vi "TDMS2TDMGlobalLog.vi"(0 "Original Name":string, 1 "New Name":string, 2 "Log File Path":path, 3 "Original Datatype":string, 4 "New Datatype":string, 5 "error in (no error)":errorcluster, 6 "Str Refnum":refnum<vi>, 8 "Operation":T1) -> (19 "error out":errorcluster)   [LabVIEW 2020]
uses:
  <vilib>/Utility/tdmsutil.llb/TDMS2TDMLogOperation.ctl
  <vilib>/Utility/error.llb/DialogType.ctl
  Instance           5 25Saved   TDMS2TDMGlobalLog .vi
  Instance           3 25Saved   TDMS2TDMGlobalLog .vi
  Instance           2 25Saved   TDMS2TDMGlobalLog .vi
  Instance           1 25Saved   TDMS2TDMGlobalLog .vi
  Instance           4 25Saved   TDMS2TDMGlobalLog .vi
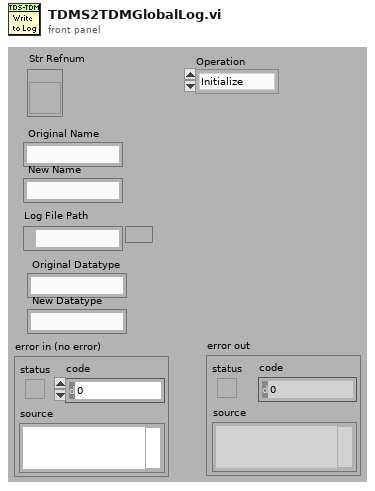
[diagram p1: front panel]
types:
  T1 = typedef "TDMS2TDMLogOperation.ctl" = enum16{"Initialize", "Data Conversion", "Name Conversion", "Write Log File"}
  T2 = enum16{"open", "replace", "create", "open or create", "replace or create", "replace or create with confirmation"}
  T3 = typedef "DialogType.ctl" = u16
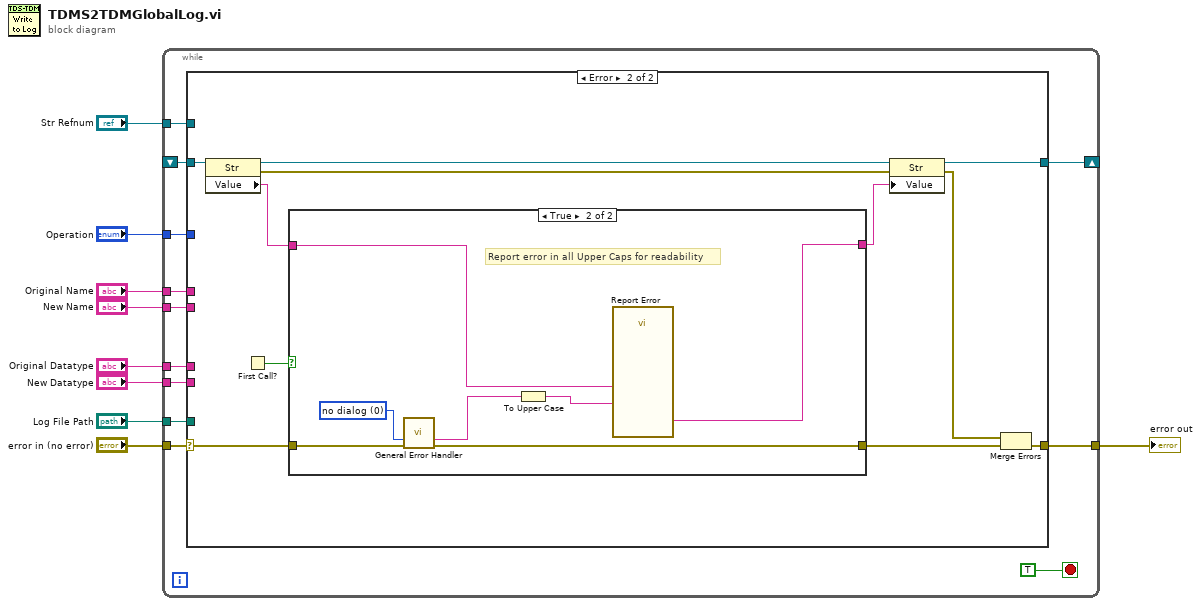
[diagram p0: block diagram]
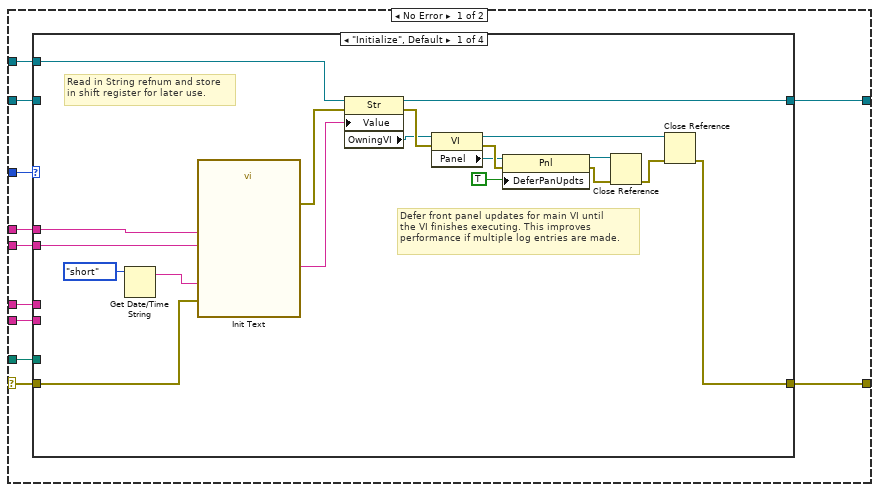
[diagram p2: hidden frame]
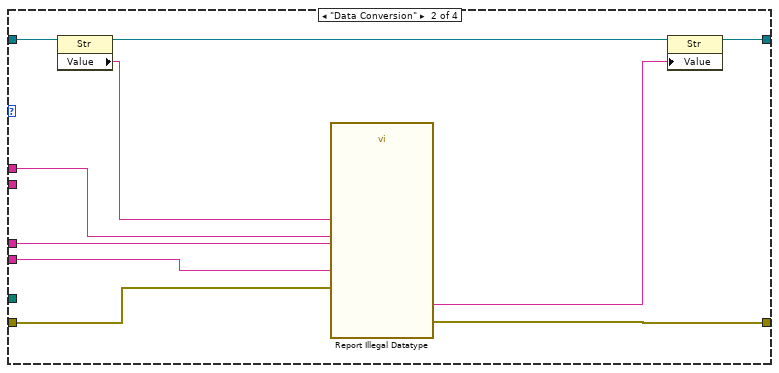
[diagram p3: hidden frame]
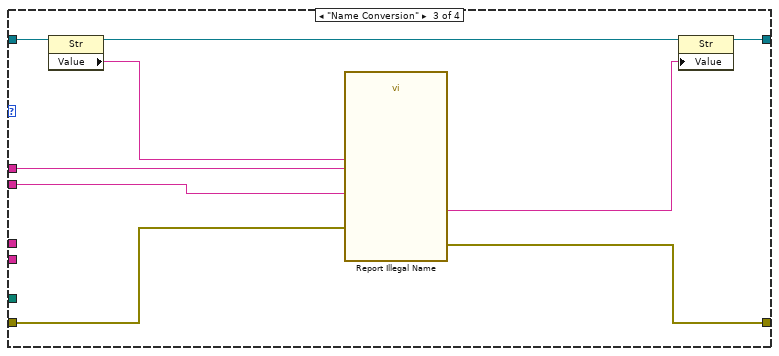
[diagram p4: hidden frame]
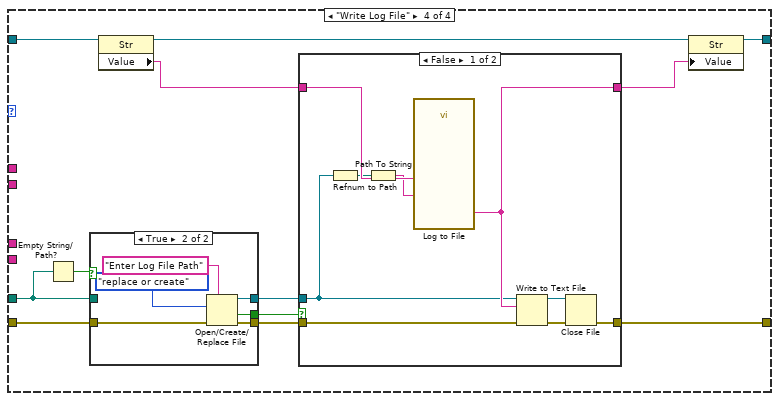
[diagram p5: hidden frame]
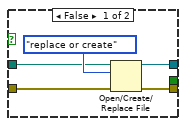
[diagram p6: hidden frame]
diagram:
  n1 = while {
    tunnel: "Operation" -> [w20]
    tunnel: "Str Refnum" -> [w19]
    shift-right: [w18] -> _
    shift-left: _ -> [w17]
    tunnel: "error in (no error)" -> [w10]
    tunnel: [w16] -> w6
    tunnel: "Log File Path" -> [w15]
    tunnel: "Original Name" -> [w14]
    tunnel: "New Name" -> [w13]
    tunnel: "Original Datatype" -> [w12]
    tunnel: "New Datatype" -> [w11]
    stop <- TRUE stop-if-true
    n2 = case shown="Error" w10 {
      selector: w10 -> [w22 w112]
      tunnel: w20 -> [w32 _]
      tunnel: w19 -> [w31 _]
      tunnel: [w30 w114] -> w18
      tunnel: w17 -> [w29 w115]
      tunnel: [w28 w107] -> w16
      tunnel: w15 -> [w27 _]
      tunnel: w14 -> [w26 _]
      tunnel: w13 -> [w25 _]
      tunnel: w12 -> [w24 _]
      tunnel: w11 -> [w23 _]
      frame No Error {
        n3 = case shown="\"Initialize\", Default" w32 {
          tunnel: w31 -> [w49 _ _ _]
          tunnel: [w48 w60 w69 w73] -> w30
          tunnel: w29 -> [_ w61 w70 w80]
          tunnel: w22 -> [w34 w54 w63 w82]
          tunnel: [w36 w52 w62 w79] -> w28
          tunnel: w27 -> [_ _ _ w72]
          tunnel: w26 -> [w47 w57 w65 _]
          tunnel: w25 -> [w35 _ w64 _]
          tunnel: w24 -> [_ w56 _ _]
          tunnel: w23 -> [_ w55 _ _]
          frame "Initialize", Default {
            # "Read in String refnum and store\nin shift register for later use."
            # "Defer front panel updates for main VI until\nthe VI finishes executing. This improves\nperformance if multiple log entries are made."
            n4 = Get Date/Time String(date format (0)=enum16{"short", "long", "abbreviated"}."short") -> (date string=w44:string)  [unwired: 2 in, 1 out]
            n5 = call "Init Text"("TDMS File"=w47, "TDM File"=w35, "Date"=w44, "error in (no error)"=w34) -> ("Result"=w46:string, "error out"=w33:errorcluster)  [unwired: 10 in]
            n6 = property class="Str"(reference=w49, error in=w33, "Value"=w46) -> (reference out=w48:refnum<vi>, error out=w51:errorcluster, "OwningVI"=w43:refnum<vi>)
            n7 = property class="VI"(reference=w43, error in=w51) -> (reference out=w38:refnum<vi>, error out=w50:errorcluster, "Panel"=w42:refnum<vi>)
            n8 = property class="Pnl"(reference=w42, error in=w50, "DeferPanUpdts"=TRUE ("Defer Panel Updates")) -> (reference out=w40:refnum<vi>, error out=w39:errorcluster)
            n9 = Close Reference(reference=w40, error in (no error)=w39) -> (error out=w37:errorcluster)
            n10 = Close Reference(reference=w38, error in (no error)=w37) -> (error out=w36:errorcluster)
          }
          frame "Data Conversion" {
            n11 = property class="Str"(reference=w61) -> (reference out=w59:refnum<vi>, "Value"=w58:string)  [unwired: 1 in, 1 out]
            n12 = call "Report Illegal Datatype"("New Datatype"=w55, "Log In"=w58, "Channel Name"=w57, "Original Datatype"=w56, "error in (no error)"=w54) -> ("Result"=w53:string, "error out"=w52:errorcluster)  [unwired: 9 in]
            n13 = property class="Str"(reference=w59, "Value"=w53) -> (reference out=w60:refnum<vi>)  [unwired: 1 in, 1 out]
          }
          frame "Name Conversion" {
            n14 = property class="Str"(reference=w70) -> (reference out=w68:refnum<vi>, "Value"=w67:string)  [unwired: 1 in, 1 out]
            n15 = call "Report Illegal Name"("Log In"=w67, "Original Name"=w65, "New Name"=w64, "error in (no error)"=w63) -> ("Result"=w66:string, "error out"=w62:errorcluster)  [unwired: 10 in]
            n16 = property class="Str"(reference=w68, "Value"=w66) -> (reference out=w69:refnum<vi>)  [unwired: 1 in, 1 out]
          }
          frame "Write Log File" {
            n17 = Empty String/Path?(string/path=w72) -> (empty?=w71:bool)
            n18 = case shown="True" w71 {
              tunnel: w82 -> [w86 w93]
              tunnel: [w85 w91] -> w81
              tunnel: [w84 w92] -> w78
              tunnel: [_ w90] -> w76
              tunnel: w72 -> [w83 _]
              frame False {
                n19 = Open/Create/Replace File(file path (use dialog)=w83, error in=w86, operation (0:open)=T2."replace or create") -> (refnum out=w84:refnum<file>, error out=w85:errorcluster)  [unwired: 3 in, 1 out]
              }
              frame True {
                n20 = Open/Create/Replace File(error in=w93, prompt="Enter Log File Path", operation (0:open)=T2."replace or create") -> (refnum out=w92:refnum<file>, cancelled=w90:bool, error out=w91:errorcluster)  [unwired: 3 in]
              }
            }
            n21 = property class="Str"(reference=w80) -> (reference out=w77:refnum<vi>, "Value"=w75:string)  [unwired: 1 in, 1 out]
            n22 = case shown="False" w76 {
              tunnel: w81 -> [w102 w104]
              tunnel: [w99 w104] -> w79
              tunnel: w78 -> [w95 _]
              tunnel: w75 -> [w98 w103]
              tunnel: [w96 w103] -> w74
              frame False {
                n23 = Refnum to Path(1:w95) -> (0:w94:path)
                n24 = Path To String(path=w94) -> (string=w97:string)
                n25 = call "Log to File"("Log In"=w98, "File Path"=w97) -> ("Result"=w96:string)  [unwired: 12 in, 1 out]
                n26 = Write to Text File(file (use dialog)=w95, text=w96, error in=w102) -> (refnum out=w101:refnum<file>, error out=w100:errorcluster)  [unwired: 1 in, 1 out]
                n27 = Close File(refnum=w101, error in=w100) -> (error out=w99:errorcluster)  [unwired: 1 out]
              }
              frame True {
              }
            }
            n28 = property class="Str"(reference=w77, "Value"=w74) -> (reference out=w73:refnum<vi>)  [unwired: 1 in, 1 out]
          }
        }
      }
      frame Error {
        n29 = property class="Str"(reference=w115) -> (reference out=w113:refnum<vi>, error out=w108:errorcluster, "Value"=w110:string)  [unwired: 1 in]
        n30 = First Call?() -> (First Call?: T/F=w111:bool)
        n31 = case shown="True" w111 {
          tunnel: w112 -> [w116 w124]
          tunnel: w110 -> [w117 w123]
          tunnel: [w117 w122] -> w109
          tunnel: [w116 w120] -> w105
          frame False {
            # "Only report first error"
          }
          frame True {
            w118 = T3 0 items=["no dialog", "OK message", "continue or stop message", "OK message + warnings", "continue/stop + warnings"] ("type of dialog (OK msg:1)")
            # "Report error in all Upper Caps for readability"
            n32 = call <vilib>:"General Error Handler.vi"("type of dialog (OK msg:1)"=w118, "error in (no error)"=w124) -> ("message"=w121:string, "error out"=w120:errorcluster)  [unwired: 9 in, 3 out]
            n33 = To Upper Case(1:w121) -> (0:w119:string)
            n34 = call "Report Error"("Log In"=w123, "Error Text"=w119) -> ("Result"=w122:string)  [unwired: 12 in, 1 out]
          }
        }
        n35 = property class="Str"(reference=w113, error in=w108, "Value"=w109) -> (reference out=w114:refnum<vi>, error out=w106:errorcluster)
        n36 = Merge Errors(w106, w105) -> (w107:errorcluster)
      }
    }
  }
  "error out" <- w6
